vi "3.%2BIDSistemaID%2BSISO.vi"() -> ()   [LabVIEW 2010]
uses:
  <vilib>/Utility/file.llb/Read From Spreadsheet File (DBL).vi
  <vilib>/addons/System Identification/Model Conversion.llb/SI Convert to State-Space Model of CDT.vi
  <vilib>/addons/Control Design/_Utility/Model Viewer.llb/Model Viewer SubVI/cd_Draw State-Space Equation (SS).vi
  <vilib>/addons/Control Design/_Model Construction/Model File IO.llb/Model File IO Subvi/cd_Write Model to File (SS).vi
  <vilib>/addons/System Identification/Parametric Estimation.llb/SI Estimate State-Space Model (SISO Array).vi
  <vilib>/addons/System Identification/Model Analysis.llb/SI Model Simulation (SISO Array).vi
panel:
  out "MODELO MATEMÁTICO PLANTA - SS":picture
  in  "nùmero de estados":i32=1
  in  "stop":bool
  out "Waveform Graph":dbl[][](graph)=[[-2.67, 1853.997, 2087.33, 2090.663, 2090.663, 2097.33, 2093.997, 2093.997, 2093.997, 2097.33, 2093.997, 857.33, 97.33, 83.997, 90.663, 93.997, 83.997, 87.33, 93.997, 90.663], [-166.61063012940264, 1790.7492530367795, 1987.1989621593734, 1957.2279393678514, 1939.890791703056, 1938.4615637891961, 1930.134134639174, 1927.776406485906, 1926.5639511296883, 1929.683064580092, 1931.5209671870887, 687.235820612786, -91.92682182294811, -68.72120107004889, -41.603445425021405, -27.76373407264424, -33.80087603938517, -27.38837763115518, -18.529043853060102, -21.566730744936933]]
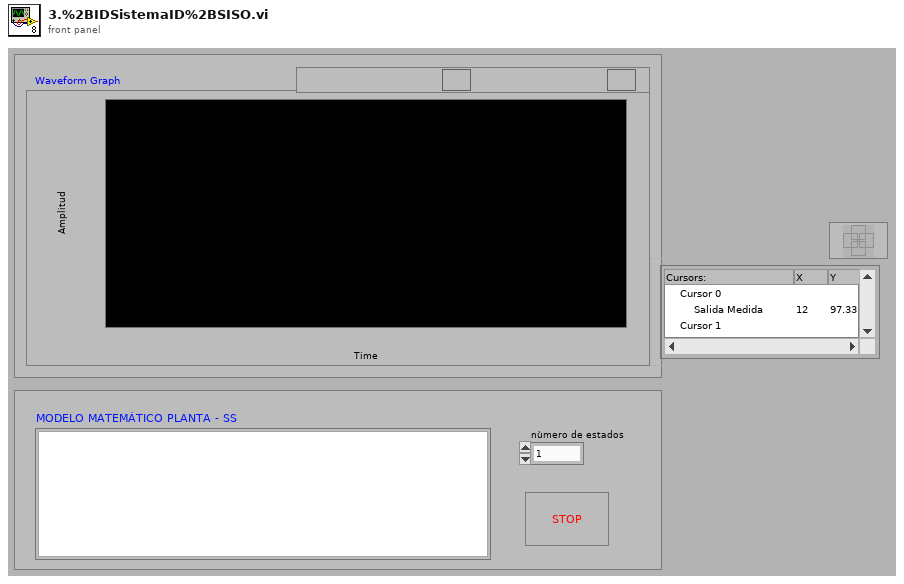
[diagram p1: front panel]
types:
  T1 = typedef "NI_SysID.lvlib/si_generic model.ctl" = cluster{"attributes":cluster{"version":string, "model type":T2, "input names":string[], "output names":string[], "notes":string}, "coefficients":cluster{"A ":dbl[][][], "B":dbl[][][], "F":dbl[][][], "C":dbl[][][], "D":dbl[][][]}, "std deviations":cluster{"A ":dbl[][][], "B":dbl[][][], "F":dbl[][][], "C":dbl[][][], "D":dbl[][][]}, "coefficients covariance":dbl[][][], "noise variance":dbl[][], "fs":dbl, "system info":cluster{"number of inputs":i32, "number of outputs":i32, "A order":i32[][], "B order":i32[][], "F order":i32[][], "C order":i32[][], "D order":i32[][], "Delays":i32[][]}, "kalman gain":dbl[][], "initial state":dbl[], "trans func":cluster{"betas":dbl[], "alphas":dbl[]}[][], "zeros-poles":cluster{"zeros":cdb[], "poles":cdb[], "gain":dbl}[][], "std of trans func":cluster{"betas":dbl[], "alphas":dbl[]}[][], "std of zeros-poles":cluster{"zeros":cdb[], "poles":cdb[], "gain":dbl}[][], "trans func (noise)":cluster{"betas":dbl[], "alphas":dbl[]}[][], "std of trans func (noise)":cluster{"betas":dbl[], "alphas":dbl[]}[][], "zeros-poles (noise)":cluster{"zeros":cdb[], "poles":cdb[], "gain":dbl}[][], "std of zeros-poles (noise)":cluster{"zeros":cdb[], "poles":cdb[], "gain":dbl}[][], "Symbolic State Space Model":cluster{"Symbolic A":string[][], "Symbolic B":string[][], "Symbolic C":string[][], "Symbolic D":string[][], "Symbolic K":string[][], "Symbolic Initial State":string[]}, "delay":dbl[][], "variables":T3, "grey trans func spec":cluster{"orders of TF model":cluster{" num order":i32, "den order":i32}, "# of zeros/poles at origin":cluster{"zeros/poles":u16, "number ":i32}, "delay initial?":bool, "gain initial?":bool}}
  T2 = typedef "NI_SysID.lvlib/SI Model Type.ctl" = u16
  T3 = typedef "NI_SysID.lvlib/si_variables.ctl" = cluster{"name":string, "initial guess":dbl, "upper limit":dbl, "lower limit":dbl, "value":dbl}[]
  T4 = typedef "NI_LinSys_Model Typedefs.lvlib/CD State Space Model (MIMO).ctl" = cluster{"properties":T5, "A":dbl[][], "B":dbl[][], "C":dbl[][], "D":dbl[][], "StateNames":string[], "Transport Delay":dbl[][]}
  T5 = typedef "NI_LinSys_Model Typedefs.lvlib/CD General Elements.ctl" = cluster{"Model name":string, "Input names":string[], "Output names":string[], "Input Delays":dbl[], "Output Delays":dbl[], "Sampling Time":dbl, "Notes":string}
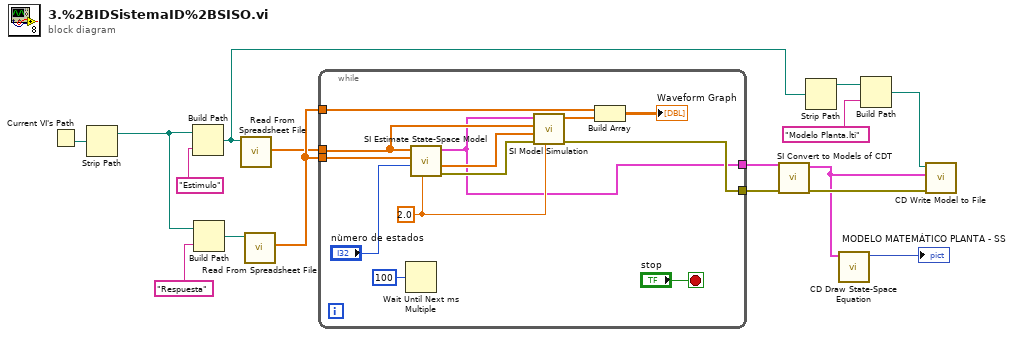
[diagram p0: block diagram]
diagram:
  n1 = Current VI's Path() -> (path=w9:path)
  n2 = Strip Path(path=w9) -> (stripped path=w1:path)  [unwired: 1 out]
  n3 = Build Path(base path=w1, name or relative path="Estimulo") -> (appended path=w2:path)
  n4 = Build Path(base path=w1, name or relative path="Respuesta") -> (appended path=w8:path)
  n5 = call-poly <vilib>:"Read From Spreadsheet File.vi"("file path (dialog if empty)"=w2) -> ("first row"=w4:dbl[])  [unwired: 3 in, 7 out]
  n6 = call-poly <vilib>:"Read From Spreadsheet File.vi"("file path (dialog if empty)"=w8) -> ("first row"=w16:dbl[])  [unwired: 3 in, 7 out]
  n7 = while {
    tunnel: w4 -> [w18]
    tunnel: w16 -> [w27]
    tunnel: w16 -> [w25]
    tunnel: [w17] -> w15
    tunnel: [w22] -> w13
    stop <- "stop" stop-if-true
    w20 = 2.0 ("sampling rate")
    n8 = Wait Until Next ms Multiple(millisecond multiple=u32 100) -> ()  [unwired: 1 out]
    n9 = call-poly <vilib>:"SI Estimate State-Space Model.vi"("sampling rate"=w20, "number of states"="nùmero de estados", "response signal"=w27, "stimulus signal"=w18) -> ("error out"=w21:errorcluster, "noise"=w23:dbl[], "system model out"=w17:T1)  [unwired: 2 in, 3 out]
    n10 = call-poly <vilib>:"SI Model Simulation.vi"("sampling rate"=w20, "error in (no error)"=w21, "noise"=w23, "stimulus signal"=w18, "system model"=w17) -> ("error out"=w22:errorcluster, "response"=w26:dbl[])  [unwired: 5 out]
    n11 = Build Array(w25, w26) -> (→"Waveform Graph":dbl[][])
  }
  n12 = call-poly <vilib>:"SI Convert to Models of CDT.vi"("error in (no error)"=w13, "system model"=w15) -> ("error out"=w14:errorcluster, "state-space model"=w3:T4)  [unwired: 1 in, 7 out]
  n13 = Strip Path(path=w2) -> (stripped path=w7:path)  [unwired: 1 out]
  n14 = call-poly <vilib>:"CD Draw State-Space Equation.vi"("State-Space Model"=w3) -> ("Equation"=→"MODELO MATEMÁTICO PLANTA - SS":picture)  [unwired: 4 in, 6 out]
  n15 = Build Path(base path=w7, name or relative path="Modelo Planta.lti") -> (appended path=w5:path)
  n16 = call-poly <vilib>:"CD Write Model to File.vi"("error in (no error)"=w14, "State-Space Model"=w3, "File Path (dialog if empty)"=w5) -> ()  [unwired: 1 in, 8 out]
